vi "SubsetTest Info Array.vi"(9 "Search Parameter  Table":string[][](array[string]), 11 "Parameter Table":string[][](array[string])) -> (3 "New Parameter Table":string[][](array[string]))   [LabVIEW 2010]
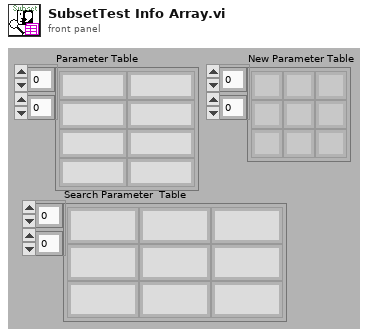
[diagram p1: front panel]
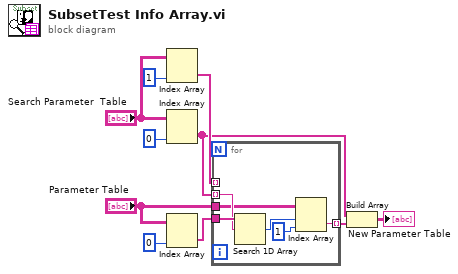
[diagram p0: block diagram]
diagram:
  n1 = Index Array(array="Search Parameter  Table", index (col)=1 ("disabled index (col)")) -> (element=w7:string[])  [unwired: 1 in]
  n2 = Index Array(array="Search Parameter  Table", index (col)=0 ("disabled index (col)")) -> (element=w3:string[])  [unwired: 1 in]
  n3 = Index Array(array="Parameter Table", index (col)=0 ("index (row)")) -> (element=w5:string[])  [unwired: 1 in]
  n4 = for {
    tunnel: w3 -> [w13] mode=indexing
    tunnel: w7 -> [_] mode=indexing
    tunnel: w5 -> [w14]
    tunnel: "Parameter Table" -> [w12]
    tunnel: [w11] -> w2 mode=indexing
    n5 = Search 1D Array(1D array=w14, element=w13) -> (index of element=w16:i32)  [unwired: 1 in]
    n6 = Index Array(array=w12, index (row)=w16, index (col)=1 ("disabled index (col)")) -> (element=w11:string)
  }
  n7 = Build Array(w3, w2) -> (→"New Parameter Table":string[][])
